vi "Set Boolean Package Attribute Value.vi"(6 "add nonexisting attribute to string (T)":bool=TRUE, 8 "error in (no error)":errorcluster, 9 "package attribute value":bool, 10 "package attribute name":string, 11 "package attributes string in":string) -> (0 "error out":errorcluster, 1 "attribute found?":bool, 2 "new attribute added to string?":bool, 3 "package attributes string out":string)   [LabVIEW 2014, in "NIPM_API.lvlib"]
doc: "Sets the value for an attribute in a package attribute string.\n\npackage attributes string in - This is the initial string containing the package attributes. For example, this string could come from reading the contents of an unpacked package's control file.\n\npackage attribute name - This is the name of the attribute whose value you want to change.\n\npackage attribute value - This is the value you want to set the attribute to.\n\nadd nonexisting attribute to string - If this VI does not find the \"package attribute name\" in the \"package attributes string in\" string, this input determines whether this VI will add the \"package attribute name\" and \"package attribute value\" to the \"package attribute string\".\nNote: If this input is TRUE, but the \"package attribute value\" is a default value (FALSE/\"no\"), then this VI will not add a new attribute to the string.\n\nnew attribute added to string? - This output will be TRUE if a new attribute (did not exist in the incoming \"package attributes string in\" string) was added to the package attributes string.\n\nattribute found? - This output will be TRUE if the \"package attribute name\" was found in the incoming \"package attributes string in\" string."
uses:
  NIPM_API.lvlib
  <vilib>/Utility/error.llb/whitespace.ctl
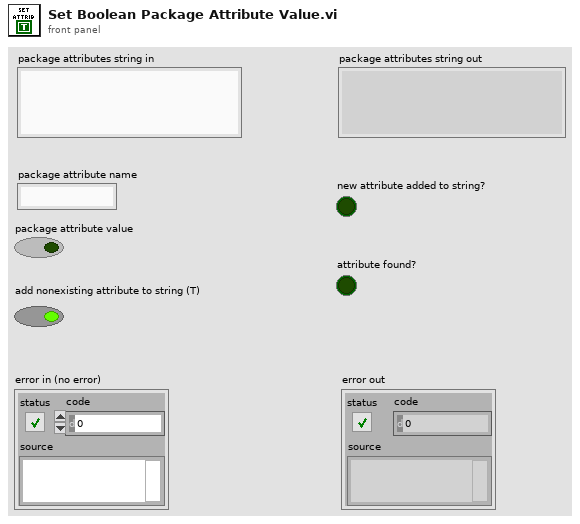
[diagram p1: front panel]
types:
  T1 = typedef "whitespace.ctl" = u16
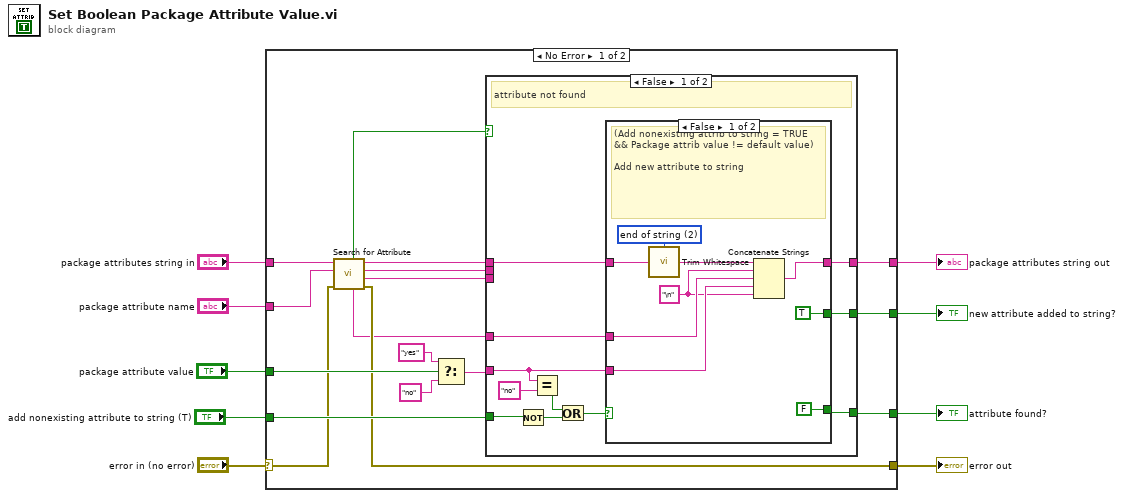
[diagram p0: block diagram]
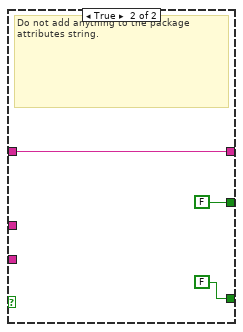
[diagram p2: hidden frame]
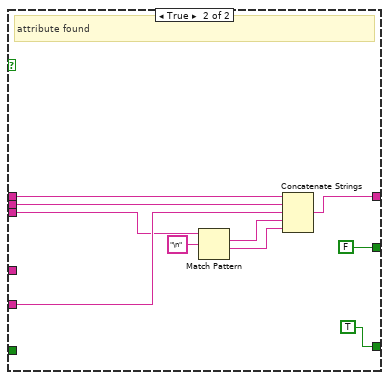
[diagram p3: hidden frame]
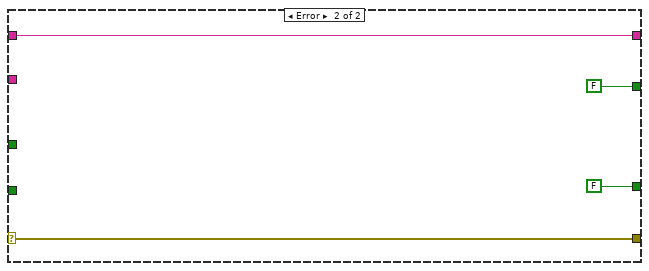
[diagram p4: hidden frame]
diagram:
  n1 = case shown="No Error" "error in (no error)" {
    selector: "error in (no error)" -> [w12 w63]
    tunnel: [w25 w60] -> w4
    tunnel: "package attribute name" -> [w17 _]
    tunnel: "package attributes string in" -> [w18 w60]
    tunnel: [w11 w63] -> w1
    tunnel: "package attribute value" -> [w26 _]
    tunnel: [w24 FALSE] -> w6
    tunnel: "add nonexisting attribute to string (T)" -> [w23 _]
    tunnel: [w22 FALSE] -> w5
    frame No Error {
      n2 = call "Search for Attribute.vi"("error in (no error)"=w12, "package attribute name"=w17, "package attributes CLI string in"=w18) -> ("error out"=w11:errorcluster, "string after attribute"=w14:string, "string matching attribute"=w15:string, "string before attribute"=w16:string, "package attribute string"=w10:string, "attribute found?"=w13:bool)  [unwired: 3 in]
      n3 = Select(t="yes", s=w26, f="no") -> (s? t:f=w21:string)
      n4 = case shown="False" w13 {
        tunnel: w16 -> [w37 w59]
        tunnel: w15 -> [_ w58]
        tunnel: w21 -> [w29 w57]
        tunnel: w14 -> [_ w56]
        tunnel: [w35 w54] -> w25
        tunnel: [w36 FALSE] -> w24
        tunnel: w10 -> [w34 _]
        tunnel: w23 -> [w31 _]
        tunnel: [w33 TRUE] -> w22
        frame False {
          # "attribute not found"
          n5 = Not(x=w31) -> (.not. x?=w32:bool)
          n6 = Equal?(x=w29, y="no") -> (x = y?=w28:bool)
          n7 = Or(x=w28, y=w32) -> (x .or. y?=w30:bool)
          n8 = case shown="False" w30 {
            tunnel: w37 -> [w46 w49]
            tunnel: [TRUE FALSE] -> w36
            tunnel: [w44 w49] -> w35
            tunnel: w34 -> [w43 _]
            tunnel: w29 -> [w42 _]
            tunnel: [FALSE FALSE] -> w33
            frame False {
              w39 = "\n"
              w40 = T1 2 items=["both", "start of string", "end of string"] ("location (both)")
              # "(Add nonexisting attrib to string = TRUE && Package attrib value != default value)\n\nAdd new attribute to string"
              n9 = call <vilib>:"Trim Whitespace.vi"("string"=w46, "location (both)"=w40) -> ("trimmed string"=w41:string)
              n10 = Concatenate Strings(w41, w39, w43, w42, w39) -> (w44:string)
            }
            frame True {
              # "Do not add anything to the package attributes string."
            }
          }
        }
        frame True {
          # "attribute found"
          n11 = Match Pattern(string=w56, regular expression="\n") -> (match substring=w52:string, after substring=w51:string)  [unwired: 1 in, 2 out]
          n12 = Concatenate Strings(w59, w58, w57, w52, w51) -> (w54:string)
        }
      }
    }
    frame Error {
    }
  }
  "error out" <- w1
  "package attributes string out" <- w4
  "new attribute added to string?" <- w6
  "attribute found?" <- w5
